vi "W7XBolo2015.vi"(1 "FPGA VI Reference In":refnum<k20>) -> (0 "FPGA VI Reference Out":refnum<k20>)   [LabVIEW 2014]
uses:
  <vilib>/Platform/TimedLoop/XDataNode/timing_clust.ctl
  <vilib>/Platform/TimedLoop/XDataNode/nitl_modes.ctl
  <vilib>/Platform/TimedLoop/XDataNode/wakeup.ctl
  <vilib>/userdefined/High Color/nirio_resource_hc.ctl
  <vilib>/FPGAPlugInAG/PCI-7813R/niLvFpga_Open_PCI-7813R.vi
  <vilib>/Utility/error.llb/Error Cluster From Error Code.vi
  <vilib>/rvi/errors/niLvFpgaAdjustHostInterfaceError.vi
  <vilib>/Utility/file.llb/Write To Spreadsheet File (DBL).vi
  <vilib>/rvi/interface/common/niFpgaWaitOnOcc.vi
  <vilib>/httpClient/POSTBuffer.vi
  <vilib>/FPGAPlugInAG/PCI-7813R/niLvFpga_Close_PCI-7813R.vi
  <vilib>/Platform/TimedLoop/XDataNode/XDataNode.xnode
  <vilib>/rvi/interface/nirviOpenFPGA/nirviOpenFPGA.xnode
  FPGA Bitfiles/W7XBolo_FPGATarget_fmain2014_Xk0NZHyrKxg.lvbitx
  f_main_2014.vi
  <vilib>/rvi/interface/nirviReadWriteControl/nirviReadWriteControl.xnode
  <vilib>/rvi/interface/nirviMethod/nirviMethod.xnode
  <vilib>/rvi/interface/nirviCloseFPGA/nirviCloseFPGA.xnode
  <vilib>/Platform/TimedLoop/XDataNode/XDNodeRunTimeDep.lvlib
  <vilib>/Analysis/NI_AALBase.lvlib
  <vilib>/httpClient/LabVIEWHTTPClient.lvlib
  NiFpgaLv.dll
  <vilib>/FPGAPlugInAG/PCI-7813R/niLvFpga_AcknowledgeIrq_PCI-7813R.vi
  <vilib>/FPGAPlugInAG/PCI-7813R/niLvFpga_ConfigureFifo_PCI-7813R.vi
  <vilib>/rvi/errors/niLvFpgaMergeErrorWithErrorCode.vi
panel:
  in  "Set Manual Time [ns]":i64
  in  "Select Timer":i32(slide) scale=0.0..2.0
  out "UTC Sample - Time":i64
  out "Frequency":u16
  in  "FreqSelRing":u16(ring) items=["0.8 ms", "1.6 ms", "3.2 ms", "6.4 ms", "12.8 ms", "19.2 ms"]
  in  "SecondFilter":bool=TRUE
  out "presamples":i32
  in  "clear?":bool
  out "UTC Time (sample0)":i64
  out "ms waited":i32=-1
  in  "start time (ms) before t=0":i32=1000
  out "Actual Depth":u32=256
  out "JSON string Offset":string
  out "body chanDesc":string="Test/raw/W7X/QSB_Bolometry/File_PARLOG/ created."
  out "headers chanDesc":string="HTTP/1.1 201 Created\r\nServer: Apache-Coyote/1.1\r\nLocation: http://archive-webapi.ipp-hgw.mpg.de/Test/raw/W7X/QSB_Bolometry/File_PARLOG/\r\nContent-Type: text/plain\r\nTransfer-Encoding: chunked\r\nDate: Wed, 15 Jul 2015 13:52:20 GMT\r\n\r\n"
  out "parms error out":errorcluster
  out "UTC Time (t=0)":i64
  in  "NSample Shot":u32=6000
  out "x-y":u32=8048
  out "Fehler READ U+P":bool
  out "TDMSDataError":errorcluster
  out "Tstart":sgl=-1.0
  out "Fehler":bool
  in  "Range001  (mV)":u8(knob)=3 scale=0.0..3.0
  in  "Range?":bool
  in  "Tab Control":T1(tab)
  in  "Tab Control 4":enum32{"1 to 64", "65 to 128"}(tab)
  out "Raw 33-64":T2
  out "Raw 1-32":T3
  out "Raw 97 - 128":T4
  out "Raw 65 - 97":T5
  in  "Tab Control 6":enum32{"1 to 64", "65 to 128"}(tab)=enum."65 to 128"
  out "Pow 33-64":T2
  out "Pow 1-32":T3
  out "Pow 97 - 128":T4
  out "Pow 65 - 96":T5
  in  "Range (mV)":enum8{"10", "20", "40", "80"}[](array[ring])=[enum."40", enum."40", enum."40", enum."40", enum."40", enum."40", enum."80", enum."80", enum."40", enum."40", enum."40", enum."80", enum."40", enum."40", enum."40", enum."80", enum."80", enum."80", enum."80", enum."80", enum."80", enum."80", enum."80", enum."80", enum."80", enum."80", enum."80", enum."80", enum."80", enum."80", enum."80", enum."80", enum."80", enum."80", enum."80", enum."80", enum."80", enum."80", enum."80", enum."80", enum."80", enum."80", enum."80", enum."80", enum."80", enum."80", enum."80", enum."80", enum."80", enum."80", enum."80", enum."80", enum."80", enum."80", enum."80", enum."80", enum."80", enum."80", enum."80", enum."80", enum."80", enum."80", enum."80", enum."80", enum."80", enum."80", enum."80", enum."80", enum."80", enum."80", enum."80", enum."80", enum."80", enum."80", enum."80", enum."80", enum."80", enum."80", enum."80", enum."80", enum."80", enum."80", enum."80", enum."80", enum."80", enum."80", enum."80", enum."80", enum."80", enum."80", enum."80", enum."80", enum."80", enum."80", enum."80", enum."80", enum."80", enum."80", enum."80", enum."80", enum."80", enum."80", enum."80", enum."80", enum."80", enum."80", enum."80", enum."80", enum."80", enum."80", enum."80", enum."80", enum."80", enum."80", enum."80", enum."80", enum."80", enum."80", enum."80", enum."80", enum."80", enum."80", enum."80", enum."80", enum."80", enum."80", enum."80", enum."80"]
  out "RangeIndex":u8[](array[numeric])
  out "DACbits 2":u16[](array[numeric])
  in  "Tab Control 2":T6(tab)=enum."33 to 64"
  out "Offset 1-32":T3
  out "Offset 33-64":T2
  out "Offset 65 - 96":T5
  out "Offset 97 - 128":T4
  out "Mean (mV)":dbl[](array[numeric]) format="%10.6f"
  out "Peak to Peak \n      (microV)":dbl[](array[numeric]) format="%10.6f"
  out "StandardDeviation\n        (microV)":dbl[](array[numeric]) format="%10.7f"
  out "RefStatus 65-96":bool[](array[boolean])
  out "RefStatus 33-64":bool[](array[boolean])
  out "RefStatus 1-32":bool[](array[boolean])
  out "RefStatus 97-128":bool[](array[boolean])
  out "MessStatus 1-32":bool[](array[boolean])
  out "MessStatus 33-64":bool[](array[boolean])
  out "MessStatus 97-128":bool[](array[boolean])
  out "MessStatus 65-96":bool[](array[boolean])
  in  "Tab Control 5":T7(tab)
  out "MessCal 17-32":T8
  out "MessCal 1-16":T9
  out "MessCal 49 - 64":T10
  out "MessCal 33 - 49":T11
  out "MessCal 81 - 96":T12
  out "MessCal 65 - 80":T13
  out "MessCal 113 - 128":T14
  out "MessCal 97 - 112":T15
  out "RMESS":dbl[](array[numeric])
  out "KappaM":dbl[](array[numeric]) format="%10.4e"
  out "TauM":dbl[](array[numeric]) format="%10.4f"
  in  "Tab Control 3":T7(tab)=enum."97 to 128"
  out "RefCal 17-32":T8
  out "RefCal 1-16":T9
  out "RefCal 49 - 64":T10
  out "RefCal 33 - 48":T11
  out "RefCal 65 - 80":T13
  out "RefCal 81 - 96":T12
  out "RefCal 113 - 128":T14
  out "RefCal 97 - 112":T15
  out "TauR":dbl[](array[numeric]) caption="TauM" format="%10.4f"
  out "KappaR":dbl[](array[numeric]) format="%10.4e"
  out "RREF":dbl[](array[numeric])
  out "Parlog error out":errorcluster
  out "Parlog error out  2":errorcluster
  out "Parlog error out  3":errorcluster
  in  "RB000":dbl[](array[numeric])
  in  "Kappa00":dbl[](array[numeric])
  in  "Tau00":dbl[](array[numeric])
  in  "Test":bool
  out "SampleTime":sgl=0.0004
  out "error out Cal":errorcluster
  out "FilterTimeOut":bool
  out "Timed Out 2":bool
  out "result":bool
  in  "stop":bool
  in  "Cancel Button":bool
  out "Acquired Samples":u32(slide) scale=-1.0..6000.0
  out "error out":errorcluster
  out "state":string="Wait for Start"
  # "Get UTC Time not working"
  # "SimpleVersionTimeOuts"
  # "FilterSelection"
types:
  T1 = enum32{"Raw", "RawOffsetFree", "Power", "Range", "Offsets", "Status", "CalibMess", "CalibRef", "Errors"}
  T2 = cluster{"Channels 33 - 40":cluster{"tstart":dbl, "FPGSampleTime":dbl, dbl[][]}, "Channels 41 - 48":cluster{"tstart":dbl, "FPGSampleTime":dbl, dbl[][]}, "Channels 49 - 56":cluster{"tstart":dbl, "FPGSampleTime":dbl, dbl[][]}, "Channels 57 - 64":cluster{"tstart":dbl, "FPGSampleTime":dbl, dbl[][]}}
  T3 = cluster{"Channels 1- 8":cluster{"tstart":dbl, "FPGSampleTime":dbl, dbl[][]}, "Channels 9 - 16":cluster{"tstart":dbl, "FPGSampleTime":dbl, dbl[][]}, "Channels 17 - 24":cluster{"tstart":dbl, "FPGSampleTime":dbl, dbl[][]}, "Channels 25 - 32":cluster{"tstart":dbl, "FPGSampleTime":dbl, dbl[][]}}
  T4 = cluster{"Channels 97 - 104":cluster{"tstart":dbl, "FPGSampleTime":dbl, dbl[][]}, "Channels 105 - 112":cluster{"tstart":dbl, "FPGSampleTime":dbl, dbl[][]}, "Channels 113 - 120":cluster{"tstart":dbl, "FPGSampleTime":dbl, dbl[][]}, "Channels 121 - 128":cluster{"tstart":dbl, "FPGSampleTime":dbl, dbl[][]}}
  T5 = cluster{"Channels 65 - 71":cluster{"tstart":dbl, "FPGSampleTime":dbl, dbl[][]}, "Channels 73 - 80":cluster{"tstart":dbl, "FPGSampleTime":dbl, dbl[][]}, "Channels 81 - 88":cluster{"tstart":dbl, "FPGSampleTime":dbl, dbl[][]}, "Channels 89- 96":cluster{"tstart":dbl, "FPGSampleTime":dbl, dbl[][]}}
  T6 = enum32{"1 to 32", "33 to 64", "65 to 96", "97 to128"}
  T7 = enum32{"1 to 32", "33 to 64", "65 to 96", "97 to 128"}
  T8 = cluster{"Channels 17 - 20":cluster{"tstart":sgl, "dt":sgl, "OutArray":dbl[][]}, "Channels 21 - 24":cluster{"tstart":sgl, "dt":sgl, "OutArray":dbl[][]}, "Channels 25 - 28":cluster{"tstart":sgl, "dt":sgl, "OutArray":dbl[][]}, "Channels 29 - 32":cluster{"tstart":sgl, "dt":sgl, "OutArray":dbl[][]}}
  T9 = cluster{"Channels 1- 4":cluster{"tstart":sgl, "dt":sgl, "OutArray":dbl[][]}, "Channels 5 - 8":cluster{"tstart":sgl, "dt":sgl, "OutArray":dbl[][]}, "Channels 9 - 12":cluster{"tstart":sgl, "dt":sgl, "OutArray":dbl[][]}, "Channels 13 - 16":cluster{"tstart":sgl, "dt":sgl, "OutArray":dbl[][]}}
  T10 = cluster{"Channels 49 - 52":cluster{"tstart":sgl, "dt":sgl, "OutArray":dbl[][]}, "Channels 53 - 56":cluster{"tstart":sgl, "dt":sgl, "OutArray":dbl[][]}, "Channels 57 - 60":cluster{"tstart":sgl, "dt":sgl, "OutArray":dbl[][]}, "Channels 61 - 64":cluster{"tstart":sgl, "dt":sgl, "OutArray":dbl[][]}}
  T11 = cluster{"Channels 33 - 36":cluster{"tstart":sgl, "dt":sgl, "OutArray":dbl[][]}, "Channels 37 - 40":cluster{"tstart":sgl, "dt":sgl, "OutArray":dbl[][]}, "Channels 41 - 44":cluster{"tstart":sgl, "dt":sgl, "OutArray":dbl[][]}, "Channels 45 - 48":cluster{"tstart":sgl, "dt":sgl, "OutArray":dbl[][]}}
  T12 = cluster{"Channels 81 - 84":cluster{"tstart":sgl, "dt":sgl, "OutArray":dbl[][]}, "Channels 85 - 88":cluster{"tstart":sgl, "dt":sgl, "OutArray":dbl[][]}, "Channels 89 - 92":cluster{"tstart":sgl, "dt":sgl, "OutArray":dbl[][]}, "Channels 93 - 96":cluster{"tstart":sgl, "dt":sgl, "OutArray":dbl[][]}}
  T13 = cluster{"Channels 65 - 68":cluster{"tstart":sgl, "dt":sgl, "OutArray":dbl[][]}, "Channels 69 - 72":cluster{"tstart":sgl, "dt":sgl, "OutArray":dbl[][]}, "Channels 73 - 76":cluster{"tstart":sgl, "dt":sgl, "OutArray":dbl[][]}, "Channels 77 - 80":cluster{"tstart":sgl, "dt":sgl, "OutArray":dbl[][]}}
  T14 = cluster{"Channels 113 - 116":cluster{"tstart":sgl, "dt":sgl, "OutArray":dbl[][]}, "Channels 117 - 120":cluster{"tstart":sgl, "dt":sgl, "OutArray":dbl[][]}, "Channels 121 - 124":cluster{"tstart":sgl, "dt":sgl, "OutArray":dbl[][]}, "Channels 125 - 128":cluster{"tstart":sgl, "dt":sgl, "OutArray":dbl[][]}}
  T15 = cluster{"Channels 97 - 100":cluster{"tstart":sgl, "dt":sgl, "OutArray":dbl[][]}, "Channels 101 - 104":cluster{"tstart":sgl, "dt":sgl, "OutArray":dbl[][]}, "Channels 104 - 108":cluster{"tstart":sgl, "dt":sgl, "OutArray":dbl[][]}, "Channels 109 - 112":cluster{"tstart":sgl, "dt":sgl, "OutArray":dbl[][]}}
  T16 = cluster{"Nchannel":i16, "ADCbits":i16, "BridgeVoltage (V)":sgl, "ExptSampleFrequency (Hz)":sgl, "CalibSampleFrequency (Hz)":sgl, "CalStep1 (V)":string, "CalStep2 (V)":string, "detector":string}[]
  T17 = cluster{"chanDescs":cluster{"name":string, "active":i32}[]}[]
  T18 = cluster{"tstart":sgl, "dt":sgl, "OutArray":dbl[][]}
  T19 = cluster{"Channels 9 - 12":cluster{"tstart":sgl, "dt":sgl, "OutArray":dbl[][]}, "Channels 9 - 12":cluster{"tstart":sgl, "dt":sgl, "OutArray":dbl[][]}, "Channels 9 - 12":cluster{"tstart":sgl, "dt":sgl, "OutArray":dbl[][]}, "Channels 9 - 12":cluster{"tstart":sgl, "dt":sgl, "OutArray":dbl[][]}}
  T20 = typedef "XDNodeRunTimeDep.lvlib/timing_clust.ctl" = cluster{"Expected End [f-1]":u64, "Actual End [f-1]":u64, "Finished Late? [f-1]":bool, "Expected End [i-1]":u64, "Actual End [i-1]":u64, "Finished Late? [i-1]":bool, "Expected Start [i]":u64, "Actual Start [i]":u64, "Expected Start [f]":u64, "Actual Start [f]":u64, "Source Name":string, "Structure Name":string, "Period":i64, "Deadline":i64, "Offset":i64, "Start":i64, "Priority":i32, "Timeout":i32, "Mode":T21, "Wakeup Reason":T22, "Error":errorcluster, "Source Type":string, "Secondary Source Type":string, "Global End Time":u64, "Global Start Time":u64, "Frame Duration":u64, "Iteration Duration":u64, "Assigned CPU":i32, "I/O Scan Engine Mode":u32}
  T21 = typedef "XDNodeRunTimeDep.lvlib/nitl_modes.ctl" = enum32{"No Change", "Process missed periods, maintain original phase", "Discard missed periods, maintain original phase", "Process missed periods, ignore original phase", "Discard missed periods, ignore original phase"}
  T22 = typedef "XDNodeRunTimeDep.lvlib/wakeup.ctl" = enum32{"Normal", "Aborted", "Asynchronous wakeup", "Timing source error", "Timed loop error", "Timeout"}
  T23 = typedef "nirio_resource_hc.ctl" = tag
  T24 = enum16{"open", "open or create", "create or replace", "create", "open (read-only)"}
  T25 = cluster{"Channels 33 - 40":cluster{"tstart":dbl, "FPGSampleTime":dbl, dbl[][]}, "Channels 41 - 48":cluster{"tstart":dbl, "FPGSampleTime":dbl, dbl[][]}, "Channels 49 - 56":cluster{"tstart":dbl, "FPGSampleTime":dbl, dbl[][]}, "Channels 57 - 58":cluster{"tstart":dbl, "FPGSampleTime":dbl, dbl[][]}}
  T26 = cluster{"Channels 1- 8":cluster{"tstart":sgl, "dt":sgl, "OutArray":dbl[][]}, "Channels 9 - 16":cluster{"tstart":sgl, "dt":sgl, "OutArray":dbl[][]}, "Channels 17 - 24":cluster{"tstart":sgl, "dt":sgl, "OutArray":dbl[][]}, "Channels 25 - 32":cluster{"tstart":sgl, "dt":sgl, "OutArray":dbl[][]}}
  T27 = cluster{"Channels 33 - 40":cluster{"tstart":sgl, "dt":sgl, "OutArray":dbl[][]}, "Channels 41 - 48":cluster{"tstart":sgl, "dt":sgl, "OutArray":dbl[][]}, "Channels 49 - 56":cluster{"tstart":sgl, "dt":sgl, "OutArray":dbl[][]}, "Channels 57 - 58":cluster{"tstart":sgl, "dt":sgl, "OutArray":dbl[][]}}
  T28 = typedef "LabVIEWHTTPClient.lvlib/ClientHandle.ctl" = refnum<k1>
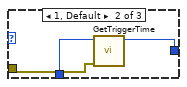
[diagram p2: hidden frame]
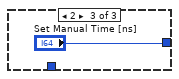
[diagram p3: hidden frame]
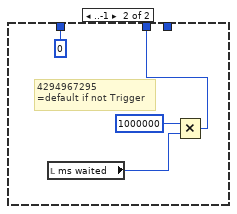
[diagram p4: hidden frame]
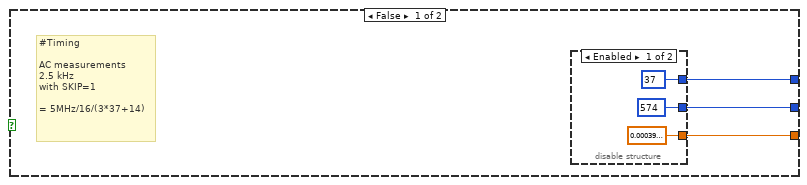
[diagram p7: hidden frame]
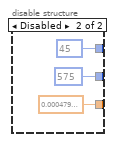
[diagram p8: hidden frame]
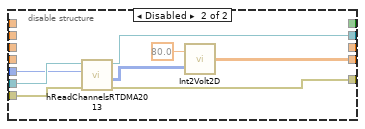
[diagram p11: hidden frame]
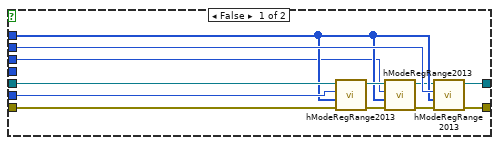
[diagram p12: hidden frame]
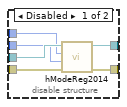
[diagram p13: hidden frame]
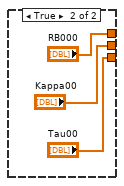
[diagram p14: hidden frame]
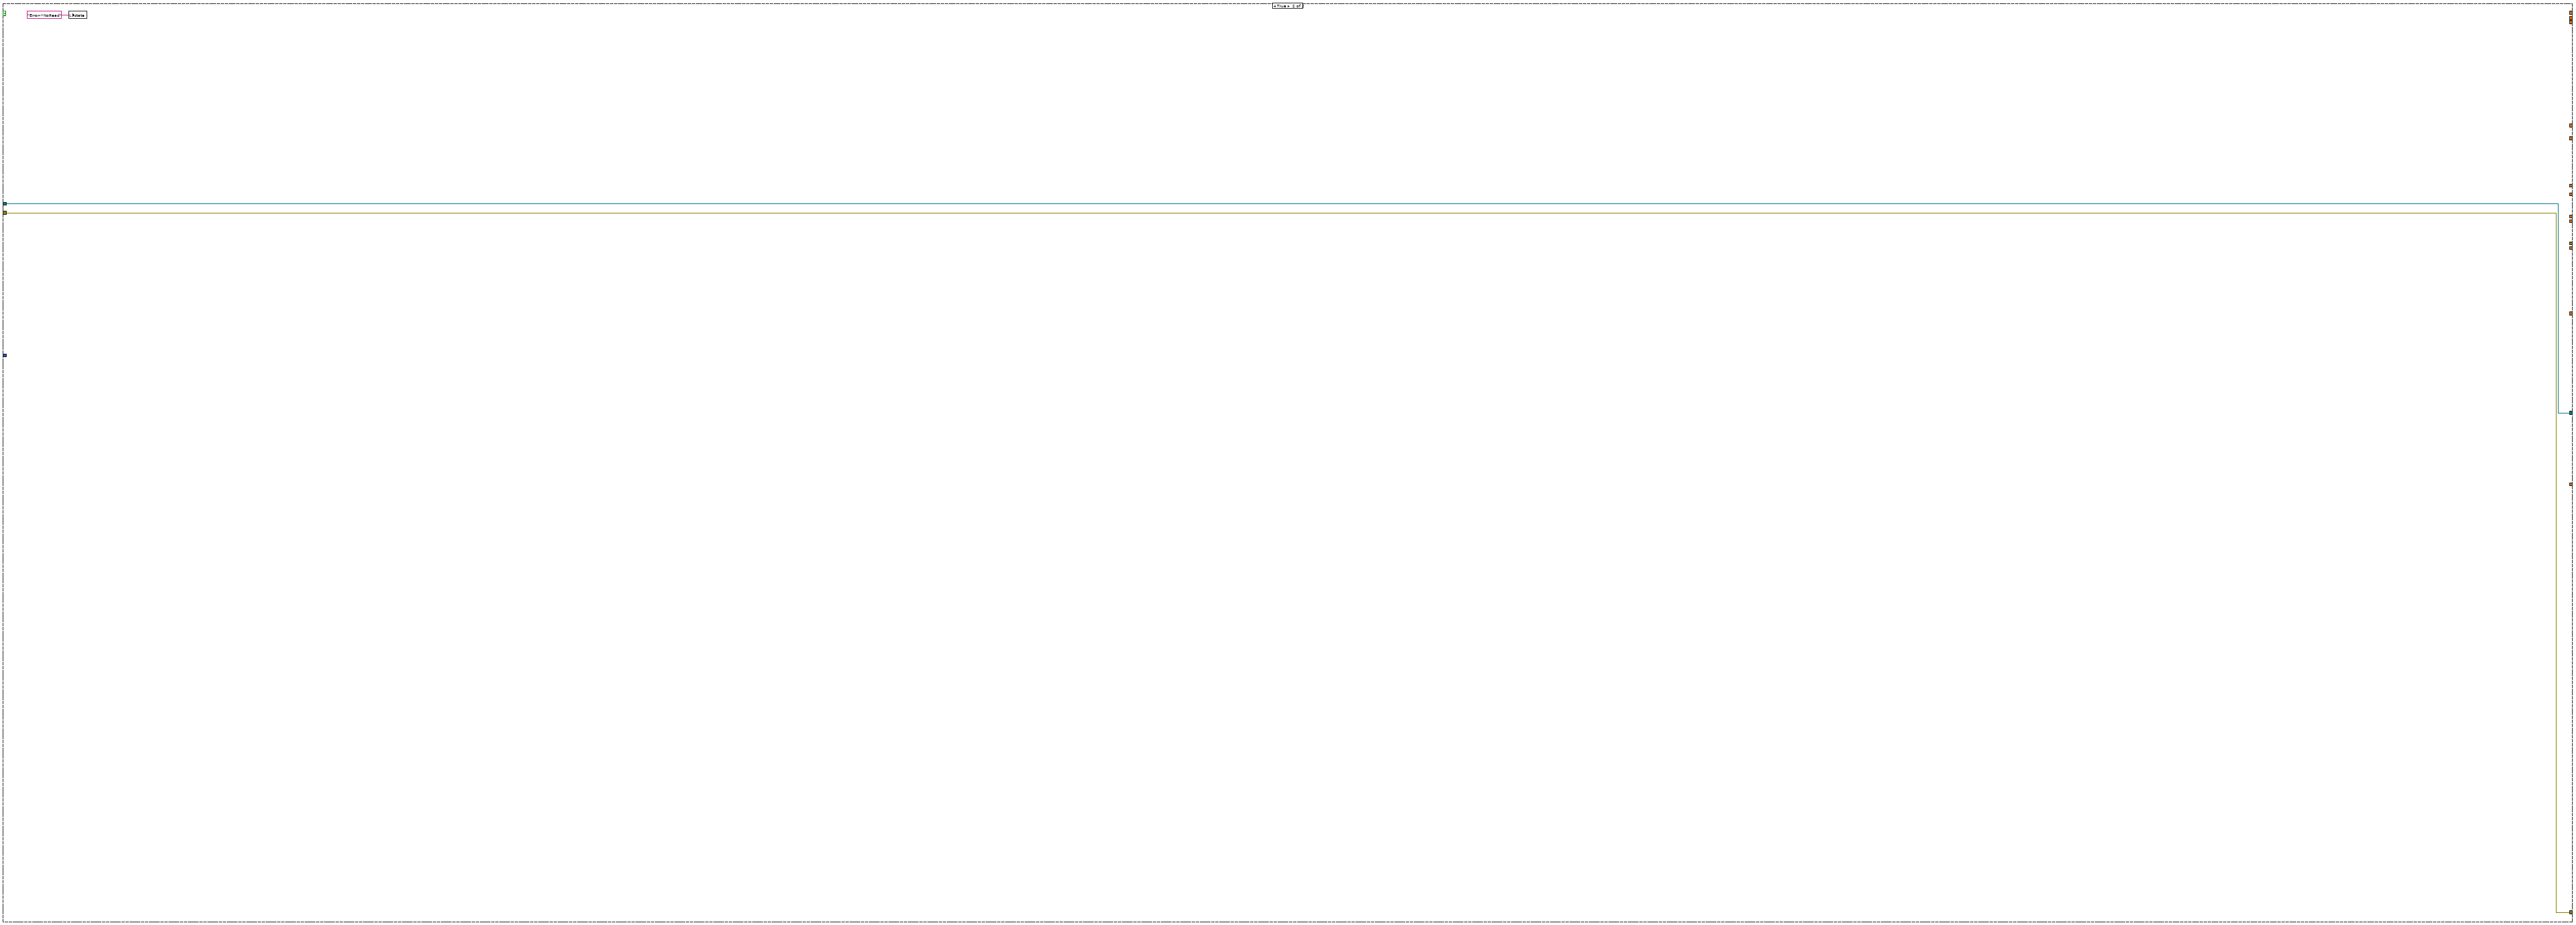
[diagram p15: hidden frame]
diagram:
  w1 = u64 400000 ("y")
  (unwired) 0.004 ("SamplePeriod")
  (unwired) 0.004 ("SamplePeriod")
  (unwired) 0.004 ("SamplePeriod")
  (unwired) 0.004 ("SamplePeriod")
  (unwired) 0.004 ("SamplePeriod")
  w47 = 1 ("sampleCount")
  w48 = 1 ("sampleCount")
  w51 = "s"  # Unit
  (unwired) u16 2500 ("SampleFrequency")
  w73 = "V"  # Unit
  (unwired) u16 2500 ("SampleFrequency")
  w79 = "A"  # Unit
  (unwired) u16 2500 ("SampleFrequency")
  w81 = "A"  # Unit
  (unwired) u16 2500 ("SampleFrequency")
  w85 = "A"  # Unit
  (unwired) u16 2500 ("SampleFrequency")
  w96 = 1 ("sampleCount")
  w100 = 1 ("sampleCount")
  w104 = 1 ("sampleCount")
  w46 = 1 ("sampleCount")
  w113 = 1 ("sampleCount")
  w120 = "Float"  # datatype
  w67 = "mV"  # Unit
  w69 = "Offset"  # label
  w138 = "Float"  # datatype
  w64 = "W"  # Unit
  w66 = "RKappa"  # label
  w140 = "Float"  # datatype
  w61 = "Ohms"  # Unit
  w63 = "RRes"  # label
  w142 = "Float"  # datatype
  w58 = "s"  # Unit
  w60 = "RTau"  # label
  w144 = "Float"  # datatype
  w55 = "W"  # Unit
  w57 = "MKappa"  # label
  w146 = "Float"  # datatype
  w54 = "Ohms"  # Unit
  w53 = "MRes"  # label
  w148 = "Float"  # datatype
  w50 = "MTau"  # label
  w150 = 10000 ("dimension size")
  w157 = 10000 ("sampleCount")
  w159 = "Float"  # datatype
  w87 = "A"  # Unit
  w89 = "BoloCalibRefFoilFit"  # label
  w160 = 10000 ("sampleCount")
  w162 = "Float"  # datatype
  w83 = "BoloCalibRefFoilCurrent"  # label
  w163 = 10000 ("sampleCount")
  w165 = "Float"  # datatype
  w75 = "BoloCalibMeasFoilFit"  # label
  w166 = 10000 ("sampleCount")
  w168 = "Float"  # datatype
  w77 = "BoloCalibMeasFoilCurrent"  # label
  w170 = 40000 ("sampleCount")
  w172 = "Float"  # datatype
  w71 = "BoloSignal"  # label
  # "Index vn dem Sample\nals der Trigger empfangen wurde"
  # "T1 Trigger\nkommt hier"
  # "A=> Internal full scale calibration\n8=> Internal zero scale calibration\nC=> System Zero scale Calibration\n2=> Continuous conversion\n\n5V reference\n80 mV scale\nChannel 1 input (voltage at bridge)\nMaster clock disable\n\np.15 7730 manual"
  # "AC 1.25 kHz Frequenz\nSKIP=0"
  n1 = flat-sequence {
    tunnel: [w233] -> w28
    tunnel: ["FPGA VI Reference In"] -> w37
    tunnel: [w234] -> w34
    tunnel: w28 -> [w234]
    frame #0 {
      n2 = Tick Count (ms)() -> (millisecond timer value=w233:u32)
    }
    frame #1 {
      n3 = case shown="True" "clear?" {
        frame False {
        }
        frame True {
          n4 = flat-sequence {
            frame #0 {
              w238 = bool[] [] ("MessStatus 1-32")
              w237 = dbl[] [] ("Kappa00")
              w241 = T18 {"tstart"=0.0, "dt"=0.0, "OutArray"=[]} ("Channels 9 - 12")
              # "Clear Graphs"
              n5 = local write "JSON string Offset"("") -> ()
              n6 = local write "MessStatus 33-64"(w238) -> ()
              n7 = local write "MessStatus 97-128"(w238) -> ()
              n8 = local write "MessStatus 1-32"(w238) -> ()
              n9 = local write "RefStatus 33-64"(w238) -> ()
              n10 = local write "RefStatus 97-128"(w238) -> ()
              n11 = local write "MessStatus 65-96"(w238) -> ()
              n12 = local write "RefStatus 1-32"(w238) -> ()
              n13 = local write "RefStatus 65-96"(w238) -> ()
              n14 = local write "StandardDeviation\n        (microV)"(w237) -> ()
              n15 = local write "Mean (mV)"(w237) -> ()
              n16 = local write "Kappa00"(w237) -> ()
              n17 = local write "KappaM"(w237) -> ()
              n18 = local write "KappaR"(w237) -> ()
              n19 = local write "TauM"(w237) -> ()
              n20 = local write "Tau00"(w237) -> ()
              n21 = local write "RMESS"(w237) -> ()
              n22 = local write "TauR"(w237) -> ()
              n23 = local write "RB000"(w237) -> ()
              n24 = local write "Peak to Peak \n      (microV)"(w237) -> ()
              n25 = local write "RREF"(w237) -> ()
              n26 = Bundle("Channels 9 - 12"=w241, "Channels 9 - 12"=w241, "Channels 9 - 12"=w241, "Channels 9 - 12"=w241) -> (w239:T19)  [unwired: 1 in]
              n27 = local write "Raw 97 - 128"(w239) -> ()
              n28 = local write "Raw 33-64"(w239) -> ()
              n29 = local write "Raw 65 - 97"(w239) -> ()
              n30 = local write "Raw 1-32"(w239) -> ()
              n31 = local write "Offset 97 - 128"(w239) -> ()
              n32 = local write "Offset 33-64"(w239) -> ()
              n33 = local write "Offset 65 - 96"(w239) -> ()
              n34 = local write "Offset 1-32"(w239) -> ()
              n35 = local write "MessCal 113 - 128"(w239) -> ()
              n36 = local write "MessCal 33 - 49"(w239) -> ()
              n37 = local write "MessCal 1-16"(w239) -> ()
              n38 = local write "MessCal 17-32"(w239) -> ()
              n39 = local write "MessCal 49 - 64"(w239) -> ()
              n40 = local write "MessCal 97 - 112"(w239) -> ()
              n41 = local write "MessCal 65 - 80"(w239) -> ()
              n42 = local write "MessCal 81 - 96"(w239) -> ()
              n43 = local write "RefCal 33 - 48"(w239) -> ()
              n44 = local write "DACbits 2"(w237) -> ()
              n45 = local write "RangeIndex"(w237) -> ()
              n46 = local write "RefCal 113 - 128"(w239) -> ()
              n47 = local write "Pow 97 - 128"(w239) -> ()
              n48 = local write "RefCal 81 - 96"(w239) -> ()
              n49 = local write "Pow 65 - 96"(w239) -> ()
              n50 = local write "RefCal 65 - 80"(w239) -> ()
              n51 = local write "RefCal 97 - 112"(w239) -> ()
              n52 = local write "RefCal 17-32"(w239) -> ()
              n53 = local write "RefCal 49 - 64"(w239) -> ()
              n54 = local write "Pow 1-32"(w239) -> ()
              n55 = local write "Pow 33-64"(w239) -> ()
              n56 = local write "RefCal 1-16"(w239) -> ()
            }
            frame #1 {
              n57 = invoke class="VI" method="Abort VI"() -> ()  [unwired: 3 in, 3 out]
            }
          }
        }
      }
    }
  }
  n58 = flat-sequence {
    tunnel: "Cancel" ("name (unnamed)") -> [w251]
    tunnel: "Transferred1" ("name (unnamed)") -> [w250]
    tunnel: u32 0 -> [w249]
    tunnel: FALSE -> [w248]
    tunnel: [w247] -> w223
    tunnel: [w246] -> w222
    tunnel: [w245] -> w221
    tunnel: [w244] -> w220
    tunnel: [u32 0] -> w40
    frame #0 {
      n59 = RT FIFO Create(0:w250, 1:w249) -> (8:w244:refnum<k33>, 11:w245:errorcluster)  [unwired: 2 in, 5 out]
      n60 = RT FIFO Create(0:w251, 1:w248) -> (8:w247:refnum<k33>, 11:w246:errorcluster)  [unwired: 3 in, 4 out]
      n61 = local write "stop"(FALSE ("stop")) -> ()
    }
  }
  n62 = node-c288() -> (w215:T20)  [unwired: 1 in, 4 out]
  n63 = timed-loop {
    tunnel: w223 -> [w262]
    tunnel: w222 -> [w261]
    tunnel: w221 -> [w260]
    tunnel: w220 -> [w259]
    shift-right: [w258] -> _
    shift-left: w40 -> [w252]
    tunnel: [w257] -> w217
    tunnel: [w256] -> w216
    tunnel: [w255] -> w219
    tunnel: [w254] -> w218
    timing: w215 -> [_]
    timing-out: [_] -> w214
    stop <- "stop" stop-if-true
    n64 = RT FIFO Read(0:w259, 1:w252, 3:w260) -> (8:w255:refnum<k33>, 9:w258:u32, 11:w254:errorcluster)  [unwired: 3 out]
    n65 = RT FIFO Write(0:w262, 1:"Cancel Button", 3:w261) -> (8:w257:refnum<k33>, 11:w256:errorcluster)  [unwired: 1 in, 3 out]
    "Acquired Samples" <- w252
  }
  n66 = node-c288(w214) -> ()  [unwired: 1 out]
  n67 = flat-sequence {
    tunnel: w219 -> [w270]
    tunnel: w218 -> [w269]
    tunnel: w217 -> [w268]
    tunnel: w216 -> [w267]
    frame #0 {
      n68 = local write "stop"(FALSE ("stop")) -> ()
      n69 = RT FIFO Delete(0:w270, 3:w269) -> ()  [unwired: 1 in, 1 out]
      n70 = RT FIFO Delete(0:w268, 3:w267) -> ()  [unwired: 1 in, 1 out]
    }
  }
  n71 = Not A Number/Path/Refnum?(number/path/refnum=w37) -> (NaN/Path/Refnum?=w36:bool)
  n72 = case shown="True" w36 {
    tunnel: [w271 w273] -> w191
    tunnel: [_ w272] -> w190
    tunnel: w37 -> [w271 _]
    frame False {
    }
    frame True {
      n73 = xnode "Open FPGA VI Reference"("resource name"=T23 "RIO0") -> ("FPGA VI Reference Out"=w273:refnum<k20>, "error out"=w272:errorcluster)  [unwired: 1 in]
    }
  }
  "error out" <- w190
  n74 = xnode "Read/Write Control"("FPGA VI Reference In"=w191, "error in"=w190, "cancel"=TRUE ("clrFifo"), "Test"=FALSE) -> ("FPGA VI Reference Out"=w232:refnum<k20>, "error out"=w231:errorcluster)
  n75 = flat-sequence {
    tunnel: w232 -> [w281]
    tunnel: w231 -> [w280]
    tunnel: [w279] -> w230
    tunnel: [w278] -> w229
    frame #0 {
      n76 = Wait (ms)(milliseconds to wait=u32 100) -> ()  [unwired: 1 out]
      n77 = xnode "Invoke Method"("FPGA VI Reference In"=w281, "error in"=w280, "IRQ Number(s)"=i32[] [0, 1, 2, 3]) -> ("FPGA VI Reference Out"=w279:refnum<k20>, "error out"=w278:errorcluster)
      "state" <- "Start" ("state")
    }
  }
  n78 = flat-sequence {
    tunnel: w229 -> [w283]
    tunnel: [w282] -> w211
    tunnel: w230 -> [w284]
    tunnel: [w285] -> w193
    frame #0 {
      n79 = local write "state"("Reset" ("state")) -> ()
      n80 = call "hReset2014.vi"("error in"=w283, "FPGA VI Reference In"=w284) -> ("error out"=w282:errorcluster, "FPGA VI Reference Out"=w285:refnum<k20>)  [unwired: 4 in]
    }
  }
  n81 = call "hFilterReg2014.vi"("error in"=w211, "Filter Modus"=u16 61 ("t"), "Frequenz"=u8 79 ("AC 1kHz Frequenz\nSKIP=0"), "FPGA VI Reference In"=w193) -> ("error out"=w196:errorcluster, "Timed Out"=w205:bool, "FPGA VI Reference Out"=w195:refnum<k20>)  [unwired: 1 in]
  "FilterTimeOut" <- w205
  n82 = call "hModeReg2014.vi"("error in"=w196, "Mode"=u16 41144, "FPGA VI Reference In"=w195) -> ("error out"=w199:errorcluster, "Timeout"=w209:bool, "FPGA VI Reference Out"=w202:refnum<k20>)  [unwired: 2 in]
  n83 = call "hModeReg2014.vi"("error in"=w199, "Mode"=u16 32952, "FPGA VI Reference In"=w202) -> ("error out"=w198:errorcluster, "Timeout"=w210:bool, "FPGA VI Reference Out"=w201:refnum<k20>)  [unwired: 2 in]
  n84 = call "hModeReg2014.vi"("error in"=w198, "Mode"=u16 8376, "FPGA VI Reference In"=w201) -> ("error out"=w207:errorcluster, "Timeout"=w208:bool, "FPGA VI Reference Out"=w206:refnum<k20>)  [unwired: 2 in]
  n85 = Compound Arithmetic op=OR(w209, w210, w208, w205) -> (w194:bool)
  "result" <- w194
  n86 = case shown="False" w194 {
    tunnel: [w292 w769] -> w32
    tunnel: [w290 w768] -> w228
    tunnel: w206 -> [w507 w769]
    tunnel: w207 -> [w506 w768]
    tunnel: [w375 _] -> w29
    tunnel: [w324 _] -> w169
    tunnel: [w370 _] -> w155
    tunnel: [w364 _] -> w156
    tunnel: [w360 _] -> w153
    tunnel: [w357 _] -> w154
    tunnel: [w288 _] -> w38
    tunnel: [w355 _] -> w137
    tunnel: [w354 _] -> w39
    tunnel: [w353 _] -> w136
    tunnel: [w352 _] -> w135
    tunnel: [w316 _] -> w134
    tunnel: [w326 _] -> w115
    tunnel: w34 -> [w328 _]
    frame False {
      (unwired) 60000  # fixed -60sec before T1 = T0
      w340 = 15000  # fixed -15sec for T0
      w378 = 2000
      w391 = u8 125  # Frequenz
      w436 = 0.0008 ("FPGSampleTime")
      w431 = 0.0
      w480 = string[] ["RAW001", "RAW002", "RAW003", "RAW004", "RAW005", "RAW006", "RAW007", "RAW008", "RAW009", "RAW010", "RAW011", "RAW012", "RAW013", "RAW014", "RAW015", "RAW016", "RAW017", "RAW018", "RAW019", "RAW020", "RAW021", "RAW022", "RAW023", "RAW024", "RAW025", "RAW026", "RAW027", "RAW028", "RAW029", "RAW030", "RAW031", "RAW032", "RAW033", "RAW034", "RAW035", "RAW036", "RAW037", "RAW038", "RAW039", "RAW040", "RAW041", "RAW042", "RAW043", "RAW044", "RAW045", "RAW046", "RAW047", "RAW048", "RAW049", "RAW050", "RAW051", "RAW052", "RAW053", "RAW054", "RAW055", "RAW056", "RAW057", "RAW058", "RAW059", "RAW060", "RAW061", "RAW062", "RAW063", "RAW064", "RAW065", "RAW066", "RAW067", "RAW068", "RAW069", "RAW070", "RAW071", "RAW072", "RAW073", "RAW074", "RAW075", "RAW076", "RAW077", "RAW078", "RAW079", "RAW080", "RAW081", "RAW082", "RAW083", "RAW084", "RAW085", "RAW086", "RAW087", "RAW088", "RAW089", "RAW090", "RAW091", "RAW092", "RAW093", "RAW094", "RAW095", "RAW096", "RAW097", "RAW098", "RAW099", "RAW100", "RAW101", "RAW102", "RAW103", "RAW104", "RAW105", "RAW106", "RAW107", "RAW108", "RAW109", "RAW110", "RAW111", "RAW112", "RAW113", "RAW114", "RAW115", "RAW116", "RAW117", "RAW118", "RAW119", "RAW120", "RAW121", "RAW122", "RAW123", "RAW124", "RAW125", "RAW126", "RAW127", "RAW128"]  # Raw channel names
      w498 = string[] ["Tstart", "SampleTime"]  # TimeProperties
      w473 = 40.0  # Rcable
      w472 = 10.0  # Rload
      w521 = sgl 0.0004  # dt
      w522 = sgl 0.0  # tstart
      w525 = sgl 0.0004  # dt
      w526 = sgl 0.0  # tstart
      w530 = sgl 80.0 ("Scale(mV)")
      # "old time from OP1"
      # "Store raw data"
      # "#Timing \n\nAC measurements\n2.083 kHz\nwith SKIP=1 \n\n= 5MHz/16/(3*45+15)"
      # "#Calibration\n\nDC 2.5 kHz Frequenz\nSKIP=0"
      # "#Offset measurement"
      # "#Offset applied"
      # "#Start measurements"
      # "#Range for measurements"
      # "A=> Internal full scale calibration\n8=> Internal zero scale calibration\nC=> System Zero scale Calibration\n2=> Continuous conversion\n\n5V reference\nscale set separately\nChannel 1 input (voltage at bridge)\nMaster clock disable\n\np.15 7730 manual"
      # "A=> Internal full scale calibration\n8=> Internal zero scale calibration\nC=> System Zero scale Calibration\n2=> Continuous conversion\n\n2.5V reference\n80 mV scale\nChannel 2 input (voltage at shunt)\nMaster clock disable\n\np.15 7730 manual"
      n87 = flat-sequence {
        tunnel: [w610] -> w346
        tunnel: [w609] -> w344
        tunnel: w507 -> [w613]
        tunnel: w506 -> [w612]
        tunnel: w346 -> [w616]
        tunnel: [w616] -> w345
        tunnel: w344 -> [w615]
        tunnel: [w615] -> w343
        tunnel: w378 -> [w620]
        tunnel: [w619] -> w380
        tunnel: w345 -> [w622]
        tunnel: w343 -> [w621]
        tunnel: [w618] -> w379
        tunnel: [w628] -> w587
        tunnel: [w627] -> w586
        tunnel: [w626] -> w584
        tunnel: w378 -> [w624]
        tunnel: w380 -> [w630]
        tunnel: w379 -> [w629]
        frame #0 {
          n88 = call "hComRegStart2013.vi"("error in"=w612, "FPGA VI Reference In"=w613) -> ("error out"=w609:errorcluster, "Timed Out"=→"Timed Out 2":bool, "FPGA VI Reference Out"=w610:refnum<k20>)  [unwired: 3 in]
          n89 = call "Wait3"("Count(mSec)"=u32 3000) -> ()  [unwired: 1 out]
        }
        frame #1 {
        }
        frame #2 {
          n90 = call "hSync&StartSampling2013.vi"("error in"=w621, "#Samples"=w620, "FPGA VI Reference In"=w622) -> ("error out"=w619:errorcluster, "FPGA VI Reference Out"=w618:refnum<k20>)  [unwired: 1 in]
          n91 = call "Wait6"("Count(mSec)"=u32 1000) -> ()  [unwired: 1 out]
          n92 = local write "state"("SyncRun" ("state")) -> ()
        }
        frame #3 {
          n93 = call "hReadChannelsRTDMA2013.vi"("FPGA VI Reference In"=w629, "Nsamples"=w624, "error in"=w630) -> ("FPGA VI Reference Out"=w628:refnum<k20>, "Fehler"=→"Fehler":bool, "RawArray"=w626:i16[][], "error out"=w627:errorcluster)  [unwired: 2 in]
          n94 = local write "state"("ReadOffset" ("state")) -> ()
        }
      }
      n95 = property on="Acquired Samples" class="Slide (strict)"("Scale.Range:Maximum"=w378) -> ()  [unwired: 2 in, 2 out]
      n96 = call "hSoftReset2013.vi"("error in"=w586, "FPGA VI Reference In"=w587) -> ("error out"=w389:errorcluster, "FPGA VI Reference Out"=w382:refnum<k20>)  [unwired: 4 in]
      n97 = call "Int2Volt2D.vi"("IntegerArray"=w584, "Scale(mV)"=sgl 80.0) -> ("RealArray"=w427:sgl[][])
      n98 = xnode "Read/Write Control"("FPGA VI Reference In"=w382, "error in"=w389, "HIREF"=TRUE) -> ("FPGA VI Reference Out"=w385:refnum<k20>, "error out"=w384:errorcluster)
      n99 = for {
        tunnel: w427 -> [w651] mode=indexing
        tunnel: [w650] -> w424 mode=indexing
        tunnel: [w649] -> w426 mode=indexing
        tunnel: [w648] -> w425 mode=indexing
        n100 = Array Subset(array=w651, index=500, length=1000) -> (w653:sgl[])
        n101 = Array Max & Min(array=w653) -> (max value=w656:sgl, min value=w657:sgl)  [unwired: 2 out]
        n102 = Subtract(x=w656, y=w657) -> (x-y=w650:sgl)
        n103 = call <vilib>:"Std Deviation and Variance.vi"("X"=w653, "Weighting (Sample)"=enum16{"Sample", "Population"}."Population") -> ("mean"=w649:dbl, "standard deviation"=w648:dbl)  [unwired: 1 out]
      }
      n104 = Array Subset(array=w427, index (row)=0, length (row)=64, index (col)=0) -> (w441:sgl[][])  [unwired: 1 in]
      n105 = Array Subset(array=w427, index (row)=64, length (row)=64, index (col)=0) -> (w437:sgl[][])  [unwired: 1 in]
      n106 = call "Visualize_Signals64.vi"("FPGSampleTime"=w436, "tstart"=w431, "Signals"=w441) -> ("plot(Signals) 33-64"=→"Offset 33-64":T25, "plot(Signals) 1-32"=→"Offset 1-32":T3)  [unwired: 7 in]
      n107 = call "Visualize_Signals64.vi"("FPGSampleTime"=w436, "tstart"=w431, "Signals"=w437) -> ("plot(Signals) 33-64"=→"Offset 97 - 128":T25, "plot(Signals) 1-32"=→"Offset 65 - 96":T3)  [unwired: 7 in]
      n108 = call "hFilterReg2014.vi"("error in"=w384, "Filter Modus"=u16 512 ("t"), "Frequenz"=w391, "FPGA VI Reference In"=w385) -> ("error out"=w383:errorcluster, "FPGA VI Reference Out"=w386:refnum<k20>)  [unwired: 1 in, 1 out]
      n109 = Multiply(x=w426, y=1000.0 ("Scale")) -> (x*y=w326:dbl[])
      "Mean (mV)" <- w326
      n110 = Multiply(x=w425, y=1000000.0 ("Scale")) -> (x*y=→"StandardDeviation\n        (microV)":dbl[])
      n111 = Multiply(x=w424, y=1000000.0 ("Scale")) -> (x*y=→"Peak to Peak \n      (microV)":dbl[])
      n112 = call "hModeReg2014.vi"("error in"=w383, "Mode"=u16 41017, "FPGA VI Reference In"=w386) -> ("error out"=w395:errorcluster, "FPGA VI Reference Out"=w394:refnum<k20>)  [unwired: 2 in, 1 out]
      n113 = call "hModeReg2014.vi"("error in"=w395, "Mode"=u16 32825, "FPGA VI Reference In"=w394) -> ("error out"=w392:errorcluster, "FPGA VI Reference Out"=w393:refnum<k20>)  [unwired: 2 in, 1 out]
      n114 = control-ref of="Acquired Samples"() -> (w581:refnum<vi>)
      n115 = control-ref of="Cancel Button"() -> (w583:refnum<vi>)
      n116 = case shown="True" "SecondFilter" {
        tunnel: [w590 w599] -> w323
        tunnel: [w589 w597] -> w377
        tunnel: [w588 w598] -> w376
        frame False {
          # "#Timing \n\nAC measurements\n2.5 kHz\nwith SKIP=1 \n\n= 5MHz/16/(3*37+14)"
          n117 = disable-structure shown="Enabled" {
            disable-tunnel: [u16 574 ("t") u16 575 ("t")] -> w588
            disable-tunnel: [u16 37 ("frequenz") u16 45 ("frequenz")] -> w589
            disable-tunnel: [sgl 0.0004 sgl 0.00048] -> w590
            frame Enabled {
            }
            frame Disabled {
            }
          }
        }
        frame True {
          # "#Timing \n\nAC measurements\n1.25 kHz\nwith SKIP=0 \n\n= 5MHz/16/250"
          n118 = call "FreqSel.vi"("Ring"="FreqSelRing") -> ("Frequency"=w597:u16, "DLY"=w598:u16, "SampleTime"=w599:sgl)  [unwired: 1 out]
        }
      }
      "SampleTime" <- w323
      "Frequency" <- w377
      n119 = call "hModeReg2014.vi"("error in"=w392, "Mode"=u16 8249, "FPGA VI Reference In"=w393) -> ("error out"=w387:errorcluster, "FPGA VI Reference Out"=w388:refnum<k20>)  [unwired: 2 in, 1 out]
      n120 = control-ref of="state"() -> (w582:refnum<vi>)
      n121 = call "hCalRT2013.vi"("FPGA VI Reference In"=w388, "cancelbutton"=w583, "state"=w582, "Acquired Samples"=w581, "error in"=w387) -> ("FPGA VI Reference Out"=w476:refnum<k20>, "Ref"=w529:i16[][], "Meas"=w579:i16[][], "error out"=w475:errorcluster)  [unwired: 6 in, 1 out]
      "error out Cal" <- w475
      n122 = call "Int2Volt2D.vi"("IntegerArray"=w529, "Scale(mV)"=w530) -> ("RealArray"=w531:sgl[][])
      n123 = call "Int2Volt2D.vi"("IntegerArray"=w579, "Scale(mV)"=w530) -> ("RealArray"=w580:sgl[][])
      n124 = flat-sequence {
        tunnel: w476 -> [w641]
        tunnel: w475 -> [w639]
        tunnel: [w640] -> w400
        tunnel: [w638] -> w399
        tunnel: [w645] -> w350
        tunnel: [w644] -> w430
        tunnel: w400 -> [w647]
        tunnel: w399 -> [w646]
        frame #0 {
          w635 = FALSE ("RESET")
          n125 = call "Wait"("Count(mSec)"=u16 3000 ("Count(uSec)")) -> ()  [unwired: 1 out]
          n126 = local write "state"("SoftReset" ("state")) -> ()
          n127 = xnode "Read/Write Control"("FPGA VI Reference In"=w641, "error in"=w639, "RLY1"=w635, "RLY2"=w635, "HIREF"=w635, "Sprung0"=w635, "Sprung1"=w635, "ScanID"=u32 0, "Test"="Test", "RESET"=TRUE) -> ("FPGA VI Reference Out"=w640:refnum<k20>, "error out"=w638:errorcluster)
        }
        frame #1 {
          n128 = xnode "Read/Write Control"("FPGA VI Reference In"=w647, "error in"=w646, "RESET"=FALSE) -> ("FPGA VI Reference Out"=w644:refnum<k20>, "error out"=w645:errorcluster)
          n129 = call "Wait5"("Count(mSec)"=u16 1000 ("Count(uSec)")) -> ()  [unwired: 1 out]
        }
      }
      n130 = xnode "Invoke Method"("FPGA VI Reference In"=w430, "error in"=w350, "Requested Depth"=u32 256) -> ("FPGA VI Reference Out"=w351:refnum<k20>, "error out"=w349:errorcluster, "Actual Depth"=→"Actual Depth":u32)
      n131 = call "hFilterReg2014.vi"("error in"=w349, "Filter Modus"=w376, "Frequenz"=w377, "FPGA VI Reference In"=w351) -> ("error out"=w520:errorcluster, "FPGA VI Reference Out"=w519:refnum<k20>)  [unwired: 1 in, 1 out]
      n132 = case shown="True" "Range?" {
        tunnel: w520 -> [w737 w753]
        tunnel: w519 -> [w738 w752]
        tunnel: [w732 w751] -> w428
        tunnel: [w735 w743] -> w429
        tunnel: u16 41096 -> [w730 w742]
        tunnel: u16 49288 -> [w727 w744]
        tunnel: u16 8328 -> [w731 w740]
        tunnel: "Range (mV)" -> [w729 _]
        tunnel: u16 32904 -> [_ w741]
        frame False {
          n133 = call "hModeRegRange2013.vi"("error in"=w737, "RangeArray"=w729, "Mode"=w730, "FPGA VI Reference In"=w738) -> ("error out"=w734:errorcluster, "FPGA VI Reference Out"=w736:refnum<k20>)  [unwired: 1 in, 1 out]
          n134 = call "hModeRegRange2013.vi"("error in"=w734, "RangeArray"=w729, "Mode"=w727, "FPGA VI Reference In"=w736) -> ("error out"=w733:errorcluster, "FPGA VI Reference Out"=w728:refnum<k20>)  [unwired: 1 in, 1 out]
          n135 = call "hModeRegRange2013.vi"("error in"=w733, "RangeArray"=w729, "Mode"=w731, "FPGA VI Reference In"=w728) -> ("error out"=w732:errorcluster, "FPGA VI Reference Out"=w735:refnum<k20>)  [unwired: 1 in, 1 out]
        }
        frame True {
          n136 = call "hModeReg2014.vi"("error in"=w753, "Range"="Range001  (mV)", "Mode"=w742, "FPGA VI Reference In"=w752) -> ("error out"=w749:errorcluster, "FPGA VI Reference Out"=w750:refnum<k20>)  [unwired: 1 in, 1 out]
          n137 = call "hModeReg2014.vi"("error in"=w749, "Range"="Range001  (mV)", "Mode"=w741, "FPGA VI Reference In"=w750) -> ("error out"=w747:errorcluster, "FPGA VI Reference Out"=w748:refnum<k20>)  [unwired: 1 in, 1 out]
          n138 = disable-structure shown="Enabled" {
            disable-tunnel: w748 -> [w759 w761]
            disable-tunnel: w747 -> [w758 w760]
            disable-tunnel: [w757 w761] -> w746
            disable-tunnel: [w756 w760] -> w745
            disable-tunnel: w744 -> [w755 _]
            disable-tunnel: "Range001  (mV)" -> [w754 _]
            frame Disabled {
              n139 = call "hModeReg2014.vi"("error in"=w758, "Range"=w754, "Mode"=w755, "FPGA VI Reference In"=w759) -> ("error out"=w756:errorcluster, "FPGA VI Reference Out"=w757:refnum<k20>)  [unwired: 1 in, 1 out]
            }
            frame Enabled {
            }
          }
          n140 = call "hModeReg2014.vi"("error in"=w745, "Range"="Range001  (mV)", "Mode"=w740, "FPGA VI Reference In"=w746) -> ("error out"=w751:errorcluster, "FPGA VI Reference Out"=w743:refnum<k20>)  [unwired: 1 in, 1 out]
        }
      }
      n141 = disable-structure shown="Enabled" {
        disable-tunnel: w429 -> [w606 w607]
        disable-tunnel: w428 -> [w605 w608]
        disable-tunnel: "Range (mV)" -> [w604 _]
        disable-tunnel: [w603 _] -> w407
        disable-tunnel: [w602 w607] -> w402
        disable-tunnel: [w601 w608] -> w336
        frame Enabled {
          n142 = call "hDACsubtract2013.vi"("FPGA VI Reference In"=w606, "Ranges"=w604, "error in"=w605) -> ("FPGA VI Reference Out"=w602:refnum<k20>, "DACbits"=w603:u16[], "error out"=w601:errorcluster)  [unwired: 10 in]
        }
        frame Disabled {
        }
      }
      n143 = property on="Acquired Samples" class="Slide (strict)"(error in=w336, "Scale.Range:Maximum"="NSample Shot") -> (error out=w335:errorcluster)  [unwired: 1 in, 1 out]
      n144 = Subtract(x=w407, y=u16 1024 ("NSample")) -> (x-y=→"DACbits 2":u16[])
      n145 = flat-sequence {
        tunnel: w335 -> [w660]
        tunnel: w402 -> [w662]
        tunnel: [w661] -> w342
        tunnel: [w659] -> w341
        tunnel: w342 -> [w670]
        tunnel: [w670] -> w332
        tunnel: w341 -> [w669]
        tunnel: [w669] -> w330
        tunnel: w337 -> [w667]
        tunnel: w332 -> [w676]
        tunnel: [w675] -> w331
        tunnel: w330 -> [w674]
        tunnel: [w673] -> w329
        tunnel: "NSample Shot" -> [w672]
        tunnel: w331 -> [w677]
        tunnel: w329 -> [w678]
        tunnel: w328 -> [w679]
        tunnel: [w677] -> w309
        tunnel: [w678] -> w308
        tunnel: w309 -> [w685]
        tunnel: w308 -> [w684]
        tunnel: [w685] -> w307
        tunnel: [w684] -> w306
        tunnel: [w683] -> w305
        tunnel: w307 -> [w697]
        tunnel: w306 -> [w698]
        tunnel: w305 -> [w691]
        tunnel: "NSample Shot" -> [w696]
        tunnel: w303 -> [w695]
        tunnel: w302 -> [w694]
        tunnel: w301 -> [w693]
        tunnel: w300 -> [w692]
        tunnel: [w690] -> w299
        tunnel: [w691] -> w298
        tunnel: [w689] -> w297
        tunnel: [w688] -> w296
        tunnel: [w687] -> w295
        tunnel: [w686] -> w294
        tunnel: [w722] -> w290
        tunnel: [w723] -> w374
        tunnel: [w724] -> w291
        tunnel: [w725] -> w292
        tunnel: [w726] -> w404
        tunnel: w298 -> [w726]
        tunnel: w297 -> [w725]
        tunnel: w296 -> [w724]
        tunnel: w295 -> [w723]
        tunnel: w294 -> [w722]
        tunnel: [w720] -> w293
        frame #0 {
          n146 = local write "state"("Wait for Start" ("state")) -> ()
          n147 = call "Wait4"("Count(mSec)"=u32 1000) -> ()  [unwired: 1 out]
          n148 = call "hComRegStart2013.vi"("error in"=w660, "FPGA VI Reference In"=w662) -> ("error out"=w659:errorcluster, "FPGA VI Reference Out"=w661:refnum<k20>)  [unwired: 3 in, 1 out]
        }
        frame #1 {
          n149 = Tick Count (ms)() -> (millisecond timer value=w668:u32)
          n150 = Subtract(x=w667, y=w668) -> (x-y=w665:u32)
          n151 = Subtract(x=w665, y=u32 50) -> (x-y=w666:u32)
          n152 = case shown="1.." w666 {
            selector: w666 -> [_ w671]
            frame ..0 {
            }
            frame 1.. {
              n153 = Wait (ms)(milliseconds to wait=w671) -> ()  [unwired: 1 out]
            }
          }
        }
        frame #2 {
          # "takes 50 ms"
          n154 = call "hSync&StartSampling2013.vi"("error in"=w674, "#Samples"=w672, "FPGA VI Reference In"=w676) -> ("error out"=w673:errorcluster, "FPGA VI Reference Out"=w675:refnum<k20>)  [unwired: 1 in]
        }
        frame #3 {
          n155 = Tick Count (ms)() -> (millisecond timer value=w680:u32)
          n156 = Subtract(x=w680, y=w679) -> (x-y=→"ms waited":u32)
          n157 = local write "state"("SyncRun" ("state")) -> ()
        }
        frame #4 {
          n158 = call "Tick Count"() -> ("Tick Count(mSec)"=w683:u32)
        }
        frame #5 {
          n159 = disable-structure shown="Enabled" {
            disable-tunnel: w698 -> [w711 w718]
            disable-tunnel: w697 -> [w710 w719]
            disable-tunnel: w696 -> [w709 w717]
            disable-tunnel: [w708 w716] -> w689
            disable-tunnel: [w707 w715] -> w686
            disable-tunnel: [w706 _] -> w690
            disable-tunnel: w693 -> [w705 _]
            disable-tunnel: w694 -> [w704 _]
            disable-tunnel: [w703 _] -> w688
            disable-tunnel: [w702 w713] -> w687
            disable-tunnel: w695 -> [w701 _]
            disable-tunnel: w692 -> [w700 _]
            frame Enabled {
              n160 = call "hReadChannels-UandP-2013.vi"("RawScal"=w704, "SumScal"=w705, "Scale(mV)"=w700, "Tau/dt"=w701, "error in"=w711, "Nsamples"=w709, "FPGA VI Reference In"=w710) -> ("error out"=w707:errorcluster, "RawArray"=w702:sgl[][], "PowerArray"=w703:sgl[][], "FPGA VI Reference Out"=w708:refnum<k20>, "Fehler"=w706:bool)
            }
            frame Disabled {
              n161 = call "hReadChannelsRTDMA2013.vi"("FPGA VI Reference In"=w719, "Nsamples"=w717, "error in"=w718) -> ("FPGA VI Reference Out"=w716:refnum<k20>, "RawArray"=w714:i16[][], "error out"=w715:errorcluster)  [unwired: 2 in, 1 out]
              n162 = call "Int2Volt2D.vi"("IntegerArray"=w714, "Scale(mV)"=sgl 80.0) -> ("RealArray"=w713:sgl[][])
            }
          }
          n163 = local write "state"("Acquiring ..." ("state")) -> ()
        }
        frame #6 {
          n164 = local write "state"("Acquiring done" ("state")) -> ()
          n165 = call "Tick Count2"() -> ("Tick Count(mSec)"=w720:u32)
        }
      }
      n166 = Subtract(x=w340, y="start time (ms) before t=0") -> (x-y=w339:i32)
      n167 = Add(x=w328, y=w339) -> (x+y=w337:u32)
      n168 = Divide(x=w580, y=w472) -> (x/y=w361:dbl[][])
      n169 = call "CalFaktor-128.vi"("CalCurrent(t)"=w361, "Rload"=w472, "Rcable"=w473) -> ("FitData"=w356:dbl[][], "Kappa"=w288:dbl[], "Tau"=w354:dbl[], "RB01"=w355:dbl[])  [unwired: 1 out]
      "KappaM" <- w288
      n170 = Array Subset(array=w361, index (row)=0 ("index"), length (row)=96 ("length")) -> (w360:dbl[][])  [unwired: 2 in]
      n171 = local read "Test"() -> (w518:bool)
      n172 = case shown="False" w518 {
        tunnel: [w763 "RB000"] -> w474
        tunnel: [w762 "Kappa00"] -> w468
        tunnel: [w764 "Tau00"] -> w303
        tunnel: w354 -> [w764 _]
        tunnel: w355 -> [w763 _]
        tunnel: w288 -> [w762 _]
        frame False {
        }
        frame True {
        }
      }
      n173 = call "Cal(SubVI)-2013.vi"("Array"=w361, "dt"=w525, "StartChan"=64 ("ChanStart"), "tstart"=w526, "FitData"=w356) -> ("plot(Signals) 1-32"=→"MessCal 65 - 80":T26, "plot(Signals) 33-64"=→"MessCal 81 - 96":T27)  [unwired: 9 in]
      n174 = call "Cal(SubVI)-2013.vi"("Array"=w361, "dt"=w525, "StartChan"=96 ("ChanStart"), "tstart"=w526, "FitData"=w356) -> ("plot(Signals) 1-32"=→"MessCal 97 - 112":T26, "plot(Signals) 33-64"=→"MessCal 113 - 128":T27)  [unwired: 9 in]
      n175 = call "Cal(SubVI)-2013.vi"("Array"=w361, "dt"=w525, "StartChan"=32 ("ChanStart"), "tstart"=w526, "FitData"=w356) -> ("plot(Signals) 1-32"=→"MessCal 33 - 49":T26, "plot(Signals) 33-64"=→"MessCal 49 - 64":T27)  [unwired: 9 in]
      n176 = call "Cal(SubVI)-2013.vi"("Array"=w361, "dt"=w525, "StartChan"=0 ("ChanStart"), "tstart"=w526, "FitData"=w356) -> ("plot(Signals) 1-32"=→"MessCal 1-16":T26, "plot(Signals) 33-64"=→"MessCal 17-32":T27)  [unwired: 9 in]
      n177 = call "Arraylimit128.vi"("LowerLimit"=400.0, "Array Input"=w355, "UpperLimit"=2000.0) -> ("BoolArray"=w571:bool[], "ArrayOutput"=w287:dbl[])
      "RMESS" <- w287
      n178 = call "Arraylimit128.vi"("LowerLimit"=2e-05, "Array Input"=w288, "UpperLimit"=0.002) -> ("BoolArray"=w573:bool[])  [unwired: 1 out]
      n179 = call "Arraylimit128.vi"("LowerLimit"=0.001, "Array Input"=w354, "UpperLimit"=0.8) -> ("BoolArray"=w572:bool[], "ArrayOutput"=w289:dbl[])
      "TauM" <- w289
      n180 = Add(x=w473, y=w472) -> (x+y=w471:dbl)
      n181 = Multiply(x=w471, y=2.0) -> (x*y=w469:dbl)
      n182 = call "U2PCoeff.vi"("Numeric"=w469, "Kappa00"=w468, "RB000"=w474) -> ("Array"=w302:dbl[], "Array 2"=w301:dbl[])
      n183 = Compound Arithmetic op=OR(w573, w572, w571) -> (w556:bool[])
      n184 = Scale By Power Of 2(n="Range (mV)", x=sgl 10.0 ("Scale(mV)")) -> (x*2^n=w300:sgl[])
      n185 = Array Subset(array=w556, index=64, length=32) -> (→"MessStatus 65-96":bool[])
      n186 = Array Subset(array=w556, index=96, length=32) -> (→"MessStatus 97-128":bool[])
      n187 = Array Subset(array=w556, index=0, length=32) -> (→"MessStatus 1-32":bool[])
      n188 = Array Subset(array=w556, index=32, length=32) -> (→"MessStatus 33-64":bool[])
      n189 = local read "start time (ms) before t=0"() -> (w334:i32)
      n190 = Divide(x=w531, y=w472) -> (x/y=w371:dbl[][])
      n191 = Divide(x=w334, y=sgl -1000.0 ("Scale(mV)")) -> (x/y=w322:sgl)
      "Tstart" <- w322
      n192 = call "CalFaktor-128.vi"("CalCurrent(t)"=w371, "Rload"=w472, "Rcable"=w473) -> ("FitData"=w365:dbl[][], "Kappa"=w316:dbl[], "Tau"=w352:dbl[], "RB01"=w353:dbl[])  [unwired: 1 out]
      "KappaR" <- w316
      n193 = Array Subset(array=w371, index (row)=0 ("index"), length (row)=96 ("length")) -> (w370:dbl[][])  [unwired: 2 in]
      n194 = Number To Decimal String(number=128 ("Channels"), width (-)=i16 4) -> (decimal integer string=w485:string)
      n195 = TDMS Open(6:FALSE ("disable buffering? (T)"), 10:T24."create or replace" ("operation (0:open)"), 11:path "C:/BoloData/W7XData.tdms" ("file path")) -> (0:w495:errorcluster, 3:w489:refnum<k34>)  [unwired: 4 in]
      n196 = Number To Fractional String(use system decimal point (T)=FALSE, number=w323, width (-)=i16 10, precision (6)=i16 8) -> (F-format string=w499:string)
      n197 = Number To Fractional String(use system decimal point (T)=FALSE, number=w322, width (-)=i16 10, precision (6)=i16 3) -> (F-format string=w497:string)
      n198 = call "Cal(SubVI)-2013.vi"("Array"=w371, "dt"=w521, "StartChan"=0 ("ChanStart"), "tstart"=w522, "FitData"=w365) -> ("plot(Signals) 1-32"=→"RefCal 1-16":T26, "plot(Signals) 33-64"=→"RefCal 17-32":T27)  [unwired: 9 in]
      n199 = call "Cal(SubVI)-2013.vi"("Array"=w371, "dt"=w521, "StartChan"=32 ("ChanStart"), "tstart"=w522, "FitData"=w365) -> ("plot(Signals) 1-32"=→"RefCal 33 - 48":T26, "plot(Signals) 33-64"=→"RefCal 49 - 64":T27)  [unwired: 9 in]
      n200 = call "Cal(SubVI)-2013.vi"("Array"=w371, "dt"=w521, "StartChan"=64 ("ChanStart"), "tstart"=w522, "FitData"=w365) -> ("plot(Signals) 1-32"=→"RefCal 65 - 80":T26, "plot(Signals) 33-64"=→"RefCal 81 - 96":T27)  [unwired: 9 in]
      n201 = call "Cal(SubVI)-2013.vi"("Array"=w371, "dt"=w521, "StartChan"=96 ("ChanStart"), "tstart"=w522, "FitData"=w365) -> ("plot(Signals) 1-32"=→"RefCal 97 - 112":T26, "plot(Signals) 33-64"=→"RefCal 113 - 128":T27)  [unwired: 9 in]
      n202 = Array Subset(array=w365, index (row)=0 ("index"), length (row)=96 ("length")) -> (w364:dbl[][])  [unwired: 2 in]
      n203 = call "Arraylimit128.vi"("LowerLimit"=400.0, "Array Input"=w353, "UpperLimit"=2000.0) -> ("BoolArray"=w540:bool[], "ArrayOutput"=w315:dbl[])
      "RREF" <- w315
      n204 = call "Arraylimit128.vi"("LowerLimit"=2e-05, "Array Input"=w316, "UpperLimit"=0.002) -> ("BoolArray"=w538:bool[])  [unwired: 1 out]
      n205 = call "Arraylimit128.vi"("LowerLimit"=0.001, "Array Input"=w352, "UpperLimit"=0.8) -> ("BoolArray"=w539:bool[], "ArrayOutput"=w317:dbl[])
      "TauR" <- w317
      n206 = TDMS Set Properties(5:w485, 7:"Nchannels" ("DiagnosticProperties"), 8:w495, 10:"BLV" ("group name"), 11:w489) -> (0:w496:errorcluster, 2:w493:string, 3:w488:refnum<k34>)  [unwired: 2 out]
      n207 = Build Array(w497, w499) -> (w500:string[])
      n208 = TDMS Set Properties(5:w500, 7:w498, 8:w496, 10:w493, 11:w488) -> (0:w481:errorcluster, 3:w482:refnum<k34>)  [unwired: 3 out]
      n209 = Subtract(x=w293, y=w404) -> (x-y=→"x-y":u32)
      n210 = Compound Arithmetic op=OR(w538, w539, w540) -> (w555:bool[])
      n211 = Array Subset(array=w374, index (row)=0 ("index"), length (row)=96 ("length")) -> (w324:sgl[][])  [unwired: 2 in]
      n212 = Array Subset(array=w291, index (row)=64, length (row)=64, index (col)=0) -> (w457:sgl[][])  [unwired: 1 in]
      n213 = Array Subset(array=w291, index (row)=0, length (row)=64, index (col)=0) -> (w461:sgl[][])  [unwired: 1 in]
      n214 = Array Subset(array=w374, index (row)=64, length (row)=64, index (col)=0) -> (w325:sgl[][])  [unwired: 1 in]
      n215 = Array Subset(array=w374, index (row)=0, length (row)=64, index (col)=0) -> (w314:sgl[][])  [unwired: 1 in]
      n216 = Build Array(w289, w288, w287, w317, w316, w315) -> (w310:dbl[][])
      n217 = call-poly <vilib>:"Write To Spreadsheet File.vi"("transpose? (no:F)"=TRUE, "format (%.3f)"="%.12f", "2D data"=w310, "file path (dialog if empty)"=path "C:/BoloData/W7XParameter.txt" ("file path")) -> ()  [unwired: 4 in, 1 out]
      n218 = TDMS Write(0:w482, 5:"RRR" ("group name in (Untitled)"), 7:w480, 9:w374, 11:w481) -> (4:w479:refnum<k34>, 15:w478:errorcluster)  [unwired: 1 in, 2 out]
      n219 = Array Subset(array=w555, index=0, length=32) -> (→"RefStatus 1-32":bool[])
      n220 = Array Subset(array=w555, index=32, length=32) -> (→"RefStatus 33-64":bool[])
      n221 = Array Subset(array=w555, index=64, length=32) -> (→"RefStatus 65-96":bool[])
      n222 = Array Subset(array=w555, index=96, length=32) -> (→"RefStatus 97-128":bool[])
      n223 = TDMS Close(8:w478, 11:w479) -> (0:w375:errorcluster)  [unwired: 1 out]
      "TDMSDataError" <- w375
      n224 = call "Visualize_Signals64.vi"("FPGSampleTime"=w323, "tstart"=w322, "Signals"=w457) -> ("plot(Signals) 33-64"=→"Pow 97 - 128":T25, "plot(Signals) 1-32"=→"Pow 65 - 96":T3)  [unwired: 7 in]
      n225 = call "Visualize_Signals64.vi"("FPGSampleTime"=w323, "tstart"=w322, "Signals"=w461) -> ("plot(Signals) 33-64"=→"Pow 33-64":T25, "plot(Signals) 1-32"=→"Pow 1-32":T3)  [unwired: 7 in]
      n226 = call "Visualize_Signals64.vi"("FPGSampleTime"=w323, "tstart"=w322, "Signals"=w325) -> ("plot(Signals) 33-64"=→"Raw 97 - 128":T25, "plot(Signals) 1-32"=→"Raw 65 - 97":T3)  [unwired: 7 in]
      n227 = call "Visualize_Signals64.vi"("FPGSampleTime"=w323, "tstart"=w322, "Signals"=w314) -> ("plot(Signals) 33-64"=→"Raw 33-64":T25, "plot(Signals) 1-32"=→"Raw 1-32":T3)  [unwired: 7 in]
      n228 = Array Subset(array=w356, index (row)=0 ("index"), length (row)=96 ("length")) -> (w357:dbl[][])  [unwired: 2 in]
      n229 = call-poly <vilib>:"Write To Spreadsheet File.vi"("transpose? (no:F)"=TRUE, "format (%.3f)"="%.6f", "2D data"=w314, "file path (dialog if empty)"=path "C:/BoloData/W7XData.txt" ("file path")) -> ()  [unwired: 4 in, 1 out]
      "RangeIndex" <- "Range (mV)"
      "Fehler READ U+P" <- w299
    }
    frame True {
      n230 = local write "state"("Error->NoRead" ("state")) -> ()
    }
  }
  n231 = flat-sequence {
    tunnel: [w774] -> w5
    tunnel: w29 -> [w773]
    tunnel: w26 -> [w772]
    frame #0 {
      n232 = case shown="0" "Select Timer" {
        tunnel: [w776 w777 "Set Manual Time [ns]"] -> w774
        tunnel: w773 -> [w775 w779 _]
        tunnel: w772 -> [_ w778 _]
        frame 0 {
          n233 = call "Get UTC from NTP.vi"("error in (no error)"=w775) -> ("UTC Time"=w776:i64)  [unwired: 9 in, 1 out]
        }
        frame 1, Default {
          n234 = call "GetTriggerTime.vi"("error in (no error)"=w779, "TriggerIndex (1)"=w778) -> ("TriggerTime [ns]"=w777:i64)  [unwired: 8 in, 1 out]
        }
        frame 2 {
        }
      }
    }
  }
  n235 = xnode "Read/Write Control"("FPGA VI Reference In"=w32) -> ("FPGA VI Reference Out"=w31:refnum<k20>, "SampleTrigger2"=w33:u32)  [unwired: 1 in, 1 out]
  n236 = To Quad Integer(1:w33) -> (0:w19:i64)
  "presamples" <- w19
  n237 = Array Subset(array=w115, index=0, length=96) -> (w118:dbl[])
  n238 = Array Subset(array=w136, index=0, length=96) -> (w106:dbl[])
  n239 = Array Subset(array=w134, index=0, length=96) -> (w110:dbl[])
  n240 = Array Subset(array=w135, index=0, length=96) -> (w103:dbl[])
  n241 = Array Subset(array=w137, index=0, length=96) -> (w94:dbl[])
  n242 = Array Subset(array=w38, index=0, length=96) -> (w99:dbl[])
  n243 = Array Subset(array=w39, index=0, length=96) -> (w91:dbl[])
  n244 = case "Correct timebase depending on if Trigger detected" shown="Default" w19 {
    selector: w19 -> [w781 _]
    tunnel: [w783 w790] -> w35
    tunnel: [1 0] -> w26
    tunnel: w1 -> [w782 _]
    frame Default {
      w787 = i64 -1000000000  # ns per sec - presamples
      # "Input Sample Frequency"
      # "Anzahl der ns pro \nClock Cycle \nda"
      n245 = Multiply(x=w781, y=w787) -> (x*y=w786:i64)
      n246 = Divide(x=w786, y=w782) -> (x/y=w784:dbl)
      n247 = To Quad Integer(1:w784) -> (0:w783:i64)
    }
    frame ..-1 {
      # "4294967295\n=default if not Trigger"
      n248 = local read "ms waited"() -> (w789:i32)
      n249 = Multiply(x=i64 1000000, y=w789) -> (x*y=w790:i64)
    }
  }
  n250 = flat-sequence {
    tunnel: w31 -> [w797]
    tunnel: w228 -> [w795]
    tunnel: w36 -> [w794]
    frame #0 {
      n251 = case shown="True" w794 {
        tunnel: w797 -> [w798 w800]
        tunnel: w795 -> [_ w799]
        tunnel: [w798 _] -> w793
        frame False {
        }
        frame True {
          n252 = xnode "Close FPGA VI Reference"("FPGA VI Reference In"=w800, "error in"=w799) -> ()  [unwired: 1 out]
        }
      }
      "FPGA VI Reference Out" <- w793
      n253 = local write "state"("Stopped" ("state")) -> ()
      n254 = property on="stop" class="Bool (strict)"("Val(Sgnl)"=TRUE) -> ()  [unwired: 2 in, 2 out]
    }
  }
  n255 = Build Array(w118) -> (w114:dbl[][])
  n256 = Build Array(w106) -> (w107:dbl[][])
  n257 = Build Array(w110) -> (w109:dbl[][])
  n258 = Build Array(w103) -> (w102:dbl[][])
  n259 = Build Array(w94) -> (w95:dbl[][])
  n260 = Build Array(w99) -> (w98:dbl[][])
  n261 = Build Array(w91) -> (w92:dbl[][])
  n262 = Add(x=w5, y=w35) -> (x+y=w6:i64)
  "UTC Time (sample0)" <- w6
  n263 = local read "NSample Shot"() -> (w30:u32)
  n264 = Subtract(x=w6, y=w5) -> (x-y=w3:i64)
  n265 = Transpose 2D Array(2D array=w114) -> (transposed array=w112:dbl[][])
  n266 = Transpose 2D Array(2D array=w107) -> (transposed array=w105:dbl[][])
  n267 = Transpose 2D Array(2D array=w109) -> (transposed array=w111:dbl[][])
  n268 = Transpose 2D Array(2D array=w102) -> (transposed array=w101:dbl[][])
  n269 = Transpose 2D Array(2D array=w95) -> (transposed array=w93:dbl[][])
  n270 = Initialize Array(w6, w30) -> (w151:i64[])
  n271 = Initialize Array(w5, w150) -> (w149:i64[])
  n272 = Transpose 2D Array(2D array=w98) -> (transposed array=w97:dbl[][])
  n273 = To Quad Integer(1:w6) -> (0:w184:i64)
  n274 = Transpose 2D Array(2D array=w92) -> (transposed array=w90:dbl[][])
  n275 = Build Array(w6) -> (w42:i64[])
  n276 = Divide(x=w3, y=100000000.0) -> (x/y=→"UTC Sample - Time":dbl)
  n277 = for {
    N: w30 -> [_]
    shift-right: [w805] -> w27
    shift-left: w151 -> [w806]
    shift-right: [w802] -> _
    shift-left: w6 -> [w803]
    tunnel: w1 -> [w801]
    i -> [w804]
    n278 = Add(x=w803, y=w801) -> (x+y=w802:u64)
    n279 = Replace Array Subset(array=w806, new element=w803, index=w804) -> (w805:i64[])
  }
  n280 = for {
    N: w150 -> [_]
    shift-right: [w811] -> w23
    shift-left: w149 -> [w812]
    shift-right: [w808] -> _
    shift-left: w6 -> [w809]
    tunnel: w1 -> [w807]
    i -> [w810]
    n281 = Add(x=w809, y=w807) -> (x+y=w808:u64)
    n282 = Replace Array Subset(array=w812, new element=w809, index=w810) -> (w811:i64[])
  }
  n283 = call "W7X2DJSON.vi"("values"=w105, "label"=w63, "dimensionSize"=w104, "dimensions"=w42, "dimensionCount"=96, "sampleCount"=w104, "datatype"=w140) -> ("JSON string"=w62:string)  [unwired: 4 in]
  n284 = call "W7X2DJSON.vi"("values"=w111, "label"=w66, "dimensionSize"=w46, "dimensions"=w42, "dimensionCount"=96, "sampleCount"=w46, "datatype"=w138) -> ("JSON string"=w65:string)  [unwired: 4 in]
  n285 = call "W7X2DJSON.vi"("values"=w101, "label"=w60, "dimensionSize"=w100, "dimensions"=w42, "dimensionCount"=96, "sampleCount"=w100, "datatype"=w142) -> ("JSON string"=w59:string)  [unwired: 4 in]
  n286 = call "W7X2DJSON.vi"("values"=w93, "label"=w53, "dimensionSize"=w47, "dimensions"=w42, "dimensionCount"=96, "sampleCount"=w47, "datatype"=w146) -> ("JSON string"=w52:string)  [unwired: 4 in]
  n287 = call "W7X2DJSON.vi"("values"=w97, "label"=w57, "dimensionSize"=w96, "dimensions"=w42, "dimensionCount"=96, "sampleCount"=w96, "datatype"=w144) -> ("JSON string"=w56:string)  [unwired: 4 in]
  n288 = call "W7X2DJSON.vi"("values"=w90, "label"=w50, "dimensionSize"=w48, "dimensions"=w42, "dimensionCount"=96, "sampleCount"=w48, "datatype"=w148) -> ("JSON string"=w49:string)  [unwired: 4 in]
  n289 = call "W7X2DJSON.vi"("values"=w112, "label"=w69, "dimensionSize"=w113, "dimensions"=w42, "dimensionCount"=96, "sampleCount"=w113, "datatype"=w120) -> ("JSON string"=w68:string)  [unwired: 4 in]
  "JSON string Offset" <- w68
  n290 = Replace Array Subset(array=i64[] [1399090569999999999, -1] ("dimensions"), new element=w184, index=0) -> (w41:i64[])
  n291 = call <vilib>:"OpenHandle.vi"() -> ("client handle out"=w181:T28, "error out"=w180:errorcluster)  [unwired: 14 in]
  n292 = call "W7X1DPut.vi"("dimensions"=w41, "Unit"=w64, "SigJSONbuffer"=w65, "SigLabel"=w66) -> ()  [unwired: 8 in]
  n293 = call "W7X1DPut.vi"("dimensions"=w41, "Unit"=w61, "SigJSONbuffer"=w62, "SigLabel"=w63) -> ()  [unwired: 8 in]
  n294 = call "W7X1DPut.vi"("dimensions"=w41, "Unit"=w58, "SigJSONbuffer"=w59, "SigLabel"=w60) -> ()  [unwired: 8 in]
  n295 = call "W7X1DPut.vi"("dimensions"=w41, "Unit"=w54, "SigJSONbuffer"=w52, "SigLabel"=w53) -> ()  [unwired: 8 in]
  n296 = call "W7X1DPut.vi"("dimensions"=w41, "Unit"=w55, "SigJSONbuffer"=w56, "SigLabel"=w57) -> ()  [unwired: 8 in]
  n297 = call "W7X1DPut.vi"("dimensions"=w41, "Unit"=w67, "SigJSONbuffer"=w68, "SigLabel"=w69) -> ()  [unwired: 8 in]
  n298 = call "chanDescQSB.vi"("dimensions"=w41, "values"=T17 [{"chanDescs"=[{"name"="HBCm_U30_01", "active"=1}, {"name"="HBCm_U30_02", "active"=1}, {"name"="HBCm_U30_03", "active"=1}, {"name"="HBCm_U30_04", "active"=1}, {"name"="HBCm_U30_05", "active"=1}, {"name"="HBCm_U30_06", "active"=1}, {"name"="HBCm_U30_07", "active"=1}, {"name"="HBCm_U30_08", "active"=1}, {"name"="HBCm_U30_09", "active"=1}, {"name"="HBCm_U30_10", "active"=1}, {"name"="HBCm_U30_11", "active"=1}, {"name"="HBCm_U30_12", "active"=1}, {"name"="HBCm_U30_13", "active"=1}, {"name"="HBCm_U30_14", "active"=1}, {"name"="HBCm_U30_15", "active"=1}, {"name"="HBCm_U30_16", "active"=1}, {"name"="HBCm_U30_17", "active"=1}, {"name"="HBCm_U30_18", "active"=1}, {"name"="HBCm_U30_19", "active"=1}, {"name"="HBCm_U30_20", "active"=1}, {"name"="HBCm_U30_21", "active"=1}, {"name"="HBCm_U30_22", "active"=1}, {"name"="HBCm_U30_23", "active"=1}, {"name"="HBCm_U30_24", "active"=1}, {"name"="HBCm_U30_25", "active"=1}, {"name"="HBCm_U30_26", "active"=1}, {"name"="HBCm_U30_27", "active"=1}, {"name"="HBCm_U30_28", "active"=1}, {"name"="HBCm_U30_29", "active"=1}, {"name"="HBCm_U30_30", "active"=1}, {"name"="HBCm_U30_31", "active"=1}, {"name"="HBCm_U30_32", "active"=1}, {"name"="VBCm_V21_01", "active"=1}, {"name"="VBCm_V21_02", "active"=1}, {"name"="VBCm_V21_03", "active"=1}, {"name"="VBCm_V21_04", "active"=1}, {"name"="VBCm_V21_05", "active"=1}, {"name"="VBCm_V21_06", "active"=1}, {"name"="VBCm_V21_07", "active"=1}, {"name"="VBCm_V21_08", "active"=1}, {"name"="VBCm_V21_09", "active"=1}, {"name"="VBCm_V21_10", "active"=1}, {"name"="VBCm_V21_11", "active"=1}, {"name"="VBCm_V21_12", "active"=1}, {"name"="VBCm_V21_13", "active"=1}, {"name"="VBCm_V21_14", "active"=1}, {"name"="VBCm_V21_15", "active"=1}, {"name"="VBCm_V21_16", "active"=1}, {"name"="VBCm_V21_17", "active"=1}, {"name"="VBCm_V21_18", "active"=1}, {"name"="VBCm_V21_19", "active"=1}, {"name"="VBCm_V21_20", "active"=1}, {"name"="VBCm_V21_21", "active"=1}, {"name"="VBCm_V21_22", "active"=1}, {"name"="VBCm_V21_23", "active"=1}, {"name"="VBCm_V21_24", "active"=1}, {"name"="VBCm_V21_25", "active"=1}, {"name"="VBCm_V21_26", "active"=1}, {"name"="VBCm_V21_27", "active"=1}, {"name"="VBCm_V21_28", "active"=1}, {"name"="VBCm_V21_29", "active"=1}, {"name"="VBCm_V21_30", "active"=1}, {"name"="VBCm_V21_31", "active"=1}, {"name"="VBCm_V21_32", "active"=1}, {"name"="VBCm_V21_33", "active"=1}, {"name"="VBCm_V21_34", "active"=1}, {"name"="VBCm_V21_35", "active"=1}, {"name"="VBCm_V21_36", "active"=1}, {"name"="VBCm_V21_37", "active"=1}, {"name"="VBCm_V21_38", "active"=1}, {"name"="VBCm_V21_39", "active"=1}, {"name"="VBCm_V21_40", "active"=1}, {"name"="VBCs_V21_01", "active"=1}, {"name"="VBCs_V21_02", "active"=1}, {"name"="VBCs_V21_03", "active"=1}, {"name"="VBCs_V21_04", "active"=1}, {"name"="VBCs_V21_05", "active"=1}, {"name"="VBCs_V21_06", "active"=1}, {"name"="VBCs_V21_07", "active"=1}, {"name"="VBCs_V21_08", "active"=1}, {"name"="HBCs_U30_01", "active"=1}, {"name"="HBCs_U30_02", "active"=1}, {"name"="HBCs_U30_03", "active"=1}, {"name"="HBCs_U30_04", "active"=1}, {"name"="HBCs_U30_05", "active"=1}, {"name"="HBCs_U30_06", "active"=1}, {"name"="HBCs_U30_07", "active"=1}, {"name"="HBCs_U30_08", "active"=1}, {"name"="HBCs_U30_09", "active"=1}, {"name"="HBCs_U30_10", "active"=1}, {"name"="HBCs_U30_11", "active"=1}, {"name"="HBCs_U30_12", "active"=1}, {"name"="HBCs_U30_13", "active"=1}, {"name"="HBCs_U30_14", "active"=1}, {"name"="HBCs_U30_15", "active"=1}, {"name"="HBCs_U30_16", "active"=1}]}], "label"="parms") -> ()  [unwired: 1 out]
  n299 = call "W7X1DPut.vi"("dimensions"=w41, "Unit"=w51, "SigJSONbuffer"=w49, "SigLabel"=w50) -> ()  [unwired: 8 in]
  n300 = call "parmsQSB.vi"("dimensions"=w41, "values"=T16 [{"Nchannel"=96, "ADCbits"=16, "BridgeVoltage (V)"=5.0, "ExptSampleFrequency (Hz)"=2500.0, "CalibSampleFrequency (Hz)"=2500.0, "CalStep1 (V)"="2.5", "CalStep2 (V)"="3.7", "detector"="Au_Kapton"}], "label"="parms") -> ("JSON string"=w25:string)
  n301 = call <vilib>:"AddHeader.vi"("client handle"=w181, "header"="Content-Type", "value"="application/json", "error in (no error)"=w180) -> ("client handle out"=w179:T28, "error out"=w178:errorcluster)  [unwired: 10 in]
  n302 = call "W7X2DJSON.vi"("values"=w156, "label"=w75, "dimensionSize"=w163, "dimensions"=w23, "dimensionCount"=96, "sampleCount"=w163, "datatype"=w165) -> ("JSON string"=w74:string)  [unwired: 4 in]
  n303 = call "W7X2DJSON.vi"("values"=w169, "label"=w71, "dimensionSize"=w170, "dimensions"=w27, "dimensionCount"=96, "sampleCount"=w170, "datatype"=w172) -> ("JSON string"=w70:string)  [unwired: 4 in]
  n304 = call "W7X2DJSON.vi"("values"=w153, "label"=w83, "dimensionSize"=w160, "dimensions"=w23, "dimensionCount"=96, "sampleCount"=w160, "datatype"=w162) -> ("JSON string"=w82:string)  [unwired: 4 in]
  n305 = call-poly <vilib>:"POST.vi"("client handle"=w179, "url"="http://archive-webapi/Test/raw/W7X/QSB_Bolometry/File_PARLOG/", "buffer"=w25, "error in (no error)"=w178, "timeout (10000)"=400000 ("timeout for upload")) -> ("client handle out"=w183:T28, "headers"=→"headers chanDesc":string, "body"=→"body chanDesc":string, "error out"=w20:errorcluster)  [unwired: 7 in]
  n306 = call "W7X2DJSON.vi"("values"=w155, "label"=w77, "dimensionSize"=w166, "dimensions"=w23, "dimensionCount"=96, "sampleCount"=w166, "datatype"=w168) -> ("JSON string"=w76:string)  [unwired: 4 in]
  n307 = call "W7X2DJSON.vi"("values"=w154, "label"=w89, "dimensionSize"=w157, "dimensions"=w23, "dimensionCount"=96, "sampleCount"=w157, "datatype"=w159) -> ("JSON string"=w88:string)  [unwired: 4 in]
  n308 = local read "SampleTime"() -> (w8:sgl)
  n309 = local read "SampleTime"() -> (w13:sgl)
  n310 = Reciprocal(x=w13) -> (1/x=w14:sgl)
  n311 = To Unsigned Word Integer(number=w14) -> (unsigned 16bit integer=w12:u16)
  n312 = Reciprocal(x=w13) -> (1/x=w18:sgl)
  n313 = To Unsigned Word Integer(number=w18) -> (unsigned 16bit integer=w17:u16)
  n314 = Reciprocal(x=w8) -> (1/x=w11:sgl)
  n315 = call "saveToFile.vi"("SigJSONbuffer"=w25, "dimensions"=w23, "String"="File_PARLOG" ("name or relative path")) -> ("error out"=w21:errorcluster)  [unwired: 8 in]
  n316 = Reciprocal(x=w8) -> (1/x=w9:sgl)
  n317 = Reciprocal(x=w13) -> (1/x=w16:sgl)
  n318 = To Unsigned Word Integer(number=w11) -> (unsigned 16bit integer=w10:u16)
  n319 = To Unsigned Word Integer(number=w9) -> (unsigned 16bit integer=w7:u16)
  n320 = To Unsigned Word Integer(number=w16) -> (unsigned 16bit integer=w15:u16)
  n321 = call "W7X2DPut.vi"("dimensions"=w41, "pulse_length"=4.0, "Unit"=w81, "sample period"=w8, "sample rate"=w7, "SigJSONbuffer"=w74, "SigLabel"=w75) -> ("Parlog error out"=→"Parlog error out  3":errorcluster)  [unwired: 4 in]
  n322 = call "W7X2DPut.vi"("dimensions"=w41, "pulse_length"=4.0, "Unit"=w85, "sample period"=w8, "sample rate"=w10, "SigJSONbuffer"=w82, "SigLabel"=w83) -> ("Parlog error out"=→"Parlog error out  2":errorcluster)  [unwired: 4 in]
  n323 = call <vilib>:"CloseHandle.vi"("client handle"=w183, "error in (no error)"=w20) -> ("error out"=w173:errorcluster)  [unwired: 13 in]
  n324 = call "W7X2DPut.vi"("dimensions"=w41, "pulse_length"=16.0, "Unit"=w73, "sample period"=w13, "sample rate"=w12, "SigJSONbuffer"=w70, "SigLabel"=w71) -> ()  [unwired: 4 in, 1 out]
  n325 = call "W7X2DPut.vi"("dimensions"=w41, "pulse_length"=4.0, "Unit"=w79, "sample period"=w13, "sample rate"=w17, "SigJSONbuffer"=w76, "SigLabel"=w77) -> ()  [unwired: 4 in, 1 out]
  n326 = call "W7X2DPut.vi"("dimensions"=w41, "pulse_length"=4.0, "Unit"=w87, "sample period"=w8, "sample rate"=w15, "SigJSONbuffer"=w88, "SigLabel"=w89) -> ("Parlog error out"=→"Parlog error out":errorcluster)  [unwired: 4 in]
  n327 = Merge Errors(w173, w21) -> (→"parms error out":errorcluster)
  "UTC Time (t=0)" <- w5
